vi "1A Read Sensor Data.vi"(8 "error (in)":errorcluster, 9 "EStop":refnum<notifier>, 11 "VISA resource name (in)":refnum<visa-resource-name>="COM1") -> (0 "error (out)":errorcluster, 3 "VISA resource name (out)":refnum<visa-resource-name>)   [LabVIEW 2013]
doc: "This VI reads one sentence of data from the serial port associated with the WeatherStation Sensor (which must have been initialized previously using the \"1A Helper - Init Sensor.vi\"). \n\nIt reads one byte at a time, first waiting for the \"$\" (indicating the start of a sentence), then saving all bytes until a \"*ss\" is reached (the checksum, indicating the end of a sentence)."
uses:
  trunk/Software/2-Think/2 Globals/2 Global.vi
  trunk/Software/2-Think/2 Typedefs/indicator LED.ctl
panel:
  out "NMEA sentence":string
  out "Current Status":enum16{"Waiting", "Reading", "Time Out!"}(ring)
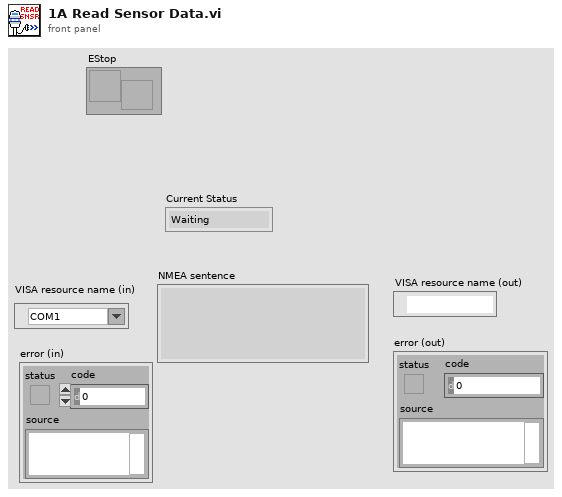
[diagram p1: front panel]
types:
  T1 = typedef "indicator LED.ctl" = bool
  T2 = typedef "generalized sensor status.ctl" = cluster{"Sensor Connected":T1, "Sensor Initialized":T1, "Sensor OK":T1, "Latest Error String":string, "GPS Lock":T1}
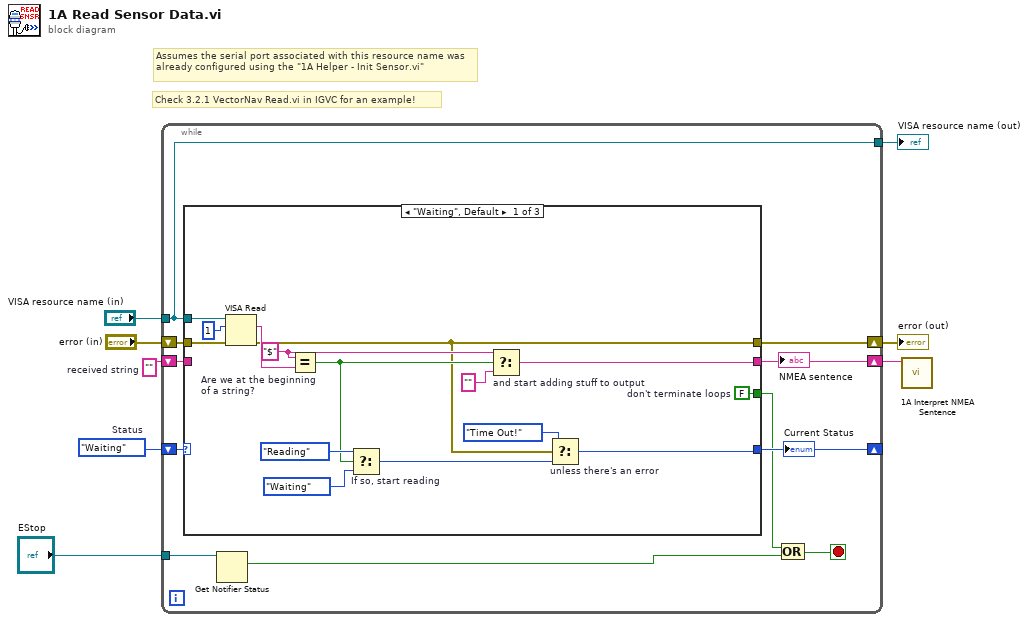
[diagram p0: block diagram]
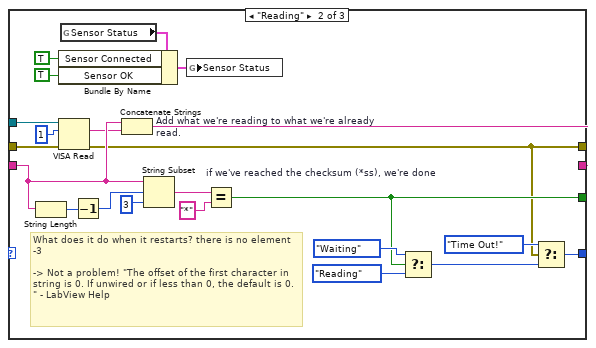
[diagram p2: hidden frame]
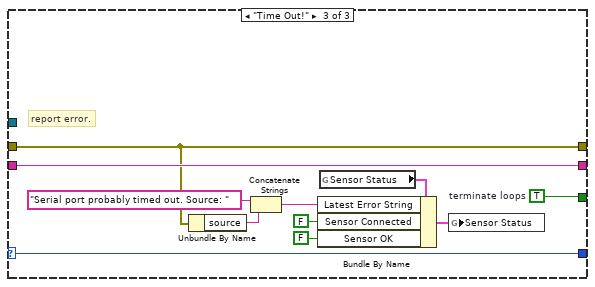
[diagram p3: hidden frame]
diagram:
  w5 = enum16{"Waiting", "Reading", "Time Out!"}."Waiting"  # Status
  w6 = ""  # received string
  # "Assumes the serial port associated with this resource name was already configured using the \"1A Helper - Init Sensor.vi\""
  # "Check 3.2.1 VectorNav Read.vi in IGVC for an example!"
  n1 = while {
    shift-right: [w12] -> w2
    shift-left: w6 -> [w19]
    shift-right: [w16] -> _
    shift-left: w5 -> [w18]
    tunnel: "VISA resource name (in)" -> [w11]
    shift-right: [w14] -> w3
    shift-left: "error (in)" -> [w15]
    tunnel: [w11] -> w4
    tunnel: "EStop" -> [w9]
    stop <- w17 stop-if-true
    n2 = case shown="\"Waiting\", Default" w18 {
      selector: w18 -> [_ _ w67]
      tunnel: w19 -> [_ w50 w66]
      tunnel: [w20 w56 w66] -> w12
      tunnel: [w25 w43 w67] -> w16
      tunnel: w11 -> [w28 w46 _]
      tunnel: w15 -> [w26 w44 w57]
      tunnel: [w23 w35 w57] -> w14
      tunnel: [w21 w40 w65] -> w13
      frame "Waiting", Default {
        w21 = FALSE  # don't terminate loops
        w30 = "$" ("x")
        n3 = VISA Read(VISA resource name=w28, byte count=u32 1, error in (no error)=w26) -> (read buffer=w29:string, error out=w23:errorcluster)  [unwired: 2 out]
        n4 = Equal? "Are we at the beginning of a string?"(x=w30, y=w29) -> (x = y?=w31:bool)
        n5 = Select "If so, start reading"(t=enum16{"Waiting", "Reading", "Time Out!"}."Reading", s=w31, f=enum16{"Waiting", "Reading", "Time Out!"}."Waiting" ("Current Status")) -> (s? t:f=w24:enum16{"Waiting", "Reading", "Time Out!"})
        n6 = Select "and start adding stuff to output"(t=w30, s=w31, f="") -> (s? t:f=w20:string)
        n7 = Select "unless there's an error"(t=enum16{"Waiting", "Reading", "Time Out!"}."Time Out!", s=w23, f=w24) -> (s? t:f=w25:enum16{"Waiting", "Reading", "Time Out!"})
      }
      frame "Reading" {
        # "What does it do when it restarts? there is no element -3\n\n-> Not a problem! \"The offset of the first character in string is 0. If unwired or if less than 0, the default is 0. \" - LabView Help"
        n8 = String Length(string=w50) -> (length=w55:i32)
        n9 = VISA Read(VISA resource name=w46, byte count=u32 1, error in (no error)=w44) -> (read buffer=w49:string, error out=w35:errorcluster)  [unwired: 2 out]
        n10 = global read "2 Global.vi" "Sensor Status"() -> (w36:T2)
        n11 = Bundle By Name(cluster=w36, "Sensor Connected"=T1 TRUE, "Sensor OK"=T1 TRUE) -> (w37:T2)
        n12 = Decrement(x=w55) -> (x-1=w54:i32)
        n13 = Concatenate Strings "Add what we're reading to what we're already read."(w50, w49) -> (w56:string)
        n14 = String Subset(string=w50, offset (0)=w54, length (rest)=3 ("length (rest)")) -> (substring=w52:string)
        n15 = global write "2 Global.vi" "Sensor Status"(w37) -> ()
        n16 = Equal? "if we've reached the checksum (*ss), we're done"(x=w52, y="*") -> (x = y?=w40:bool)
        n17 = Select(t=enum16{"Waiting", "Reading", "Time Out!"}."Waiting", s=w40, f=enum16{"Waiting", "Reading", "Time Out!"}."Reading" ("Status")) -> (s? t:f=w42:enum16{"Waiting", "Reading", "Time Out!"})
        n18 = Select(t=enum16{"Waiting", "Reading", "Time Out!"}."Time Out!", s=w35, f=w42) -> (s? t:f=w43:enum16{"Waiting", "Reading", "Time Out!"})
      }
      frame "Time Out!" {
        w65 = TRUE  # terminate loops
        # "report error."
        n19 = Unbundle By Name(w57) -> ("source"=w64:string)
        n20 = Concatenate Strings("Serial port probably timed out. Source: " ("string"), w64) -> (w63:string)
        n21 = global read "2 Global.vi" "Sensor Status"() -> (w58:T2)
        n22 = Bundle By Name(cluster=w58, "Latest Error String"=w63, "Sensor Connected"=T1 FALSE, "Sensor OK"=T1 FALSE) -> (w59:T2)
        n23 = global write "2 Global.vi" "Sensor Status"(w59) -> ()
      }
    }
    "Current Status" <- w16
    "NMEA sentence" <- w12
    n24 = Get Notifier Status(notifier=w9) -> (current notification=w10:bool)  [unwired: 1 in, 4 out]
    n25 = Compound Arithmetic op=OR(w13, w10) -> (w17:bool)
  }
  "VISA resource name (out)" <- w4
  "error (out)" <- w3
  n26 = call "1A Interpret NMEA Sentence.vi"("NMEA Sentence"=w2) -> ()  [unwired: 11 in]
